vi "Dummy_Cam.vi"(4 "Frames in sequence":u32, 6 "Image in":variant, 7 "Camera-specific in":variant, 8 "Save path":path, 9 "Capture mode":enum16{"Single frame", "Sequence"}(ring), 10 "Exposure time (s)":dbl, 11 "Operation":T2(ring)) -> (3 "Status":T1, 5 "Camera-specific out":variant)   [LabVIEW 2015]
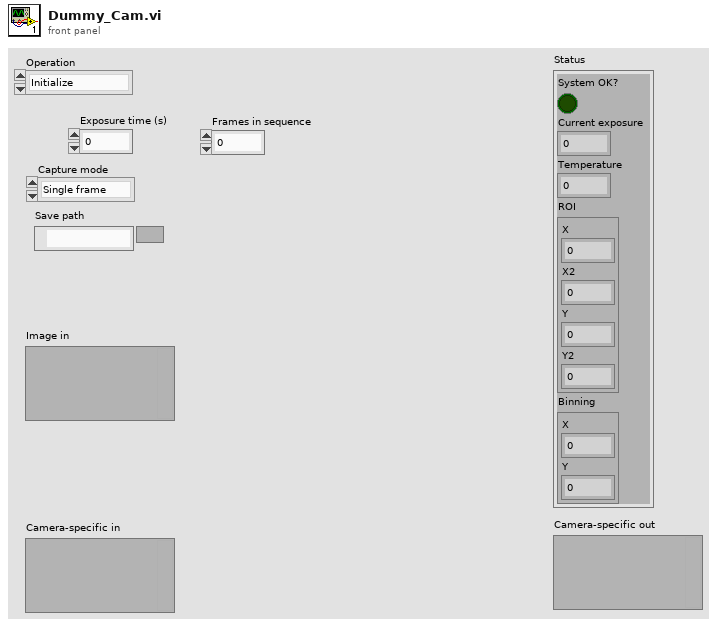
[diagram p1: front panel]
types:
  T1 = cluster{"System OK?":bool, "Current exposure":dbl, "Temperature":dbl, "ROI":cluster{"X":u32, "X2":u32, "Y":u32, "Y2":u32}, "Binning":cluster{"X":u32, "Y":u32}}
  T2 = enum16{"Initialize", "Shut down", "Set capture mode", "Set exposure", "Trigger and read", "Get status", "Other settings"}
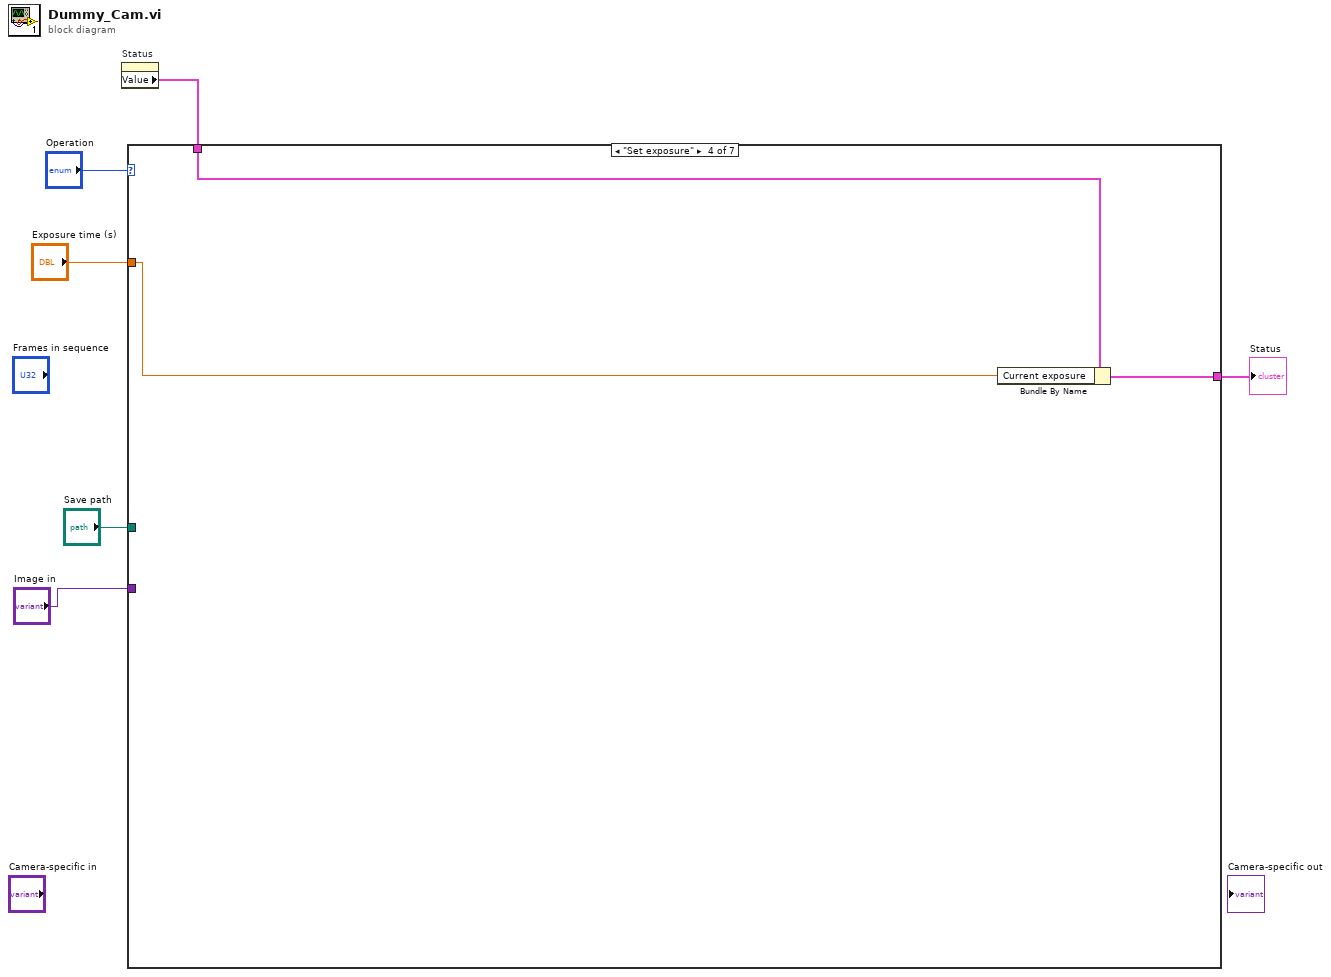
[diagram p0: block diagram]
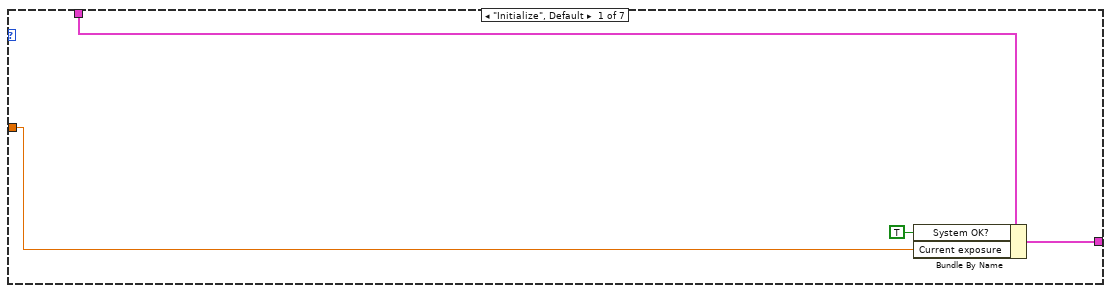
[diagram p2: hidden frame]
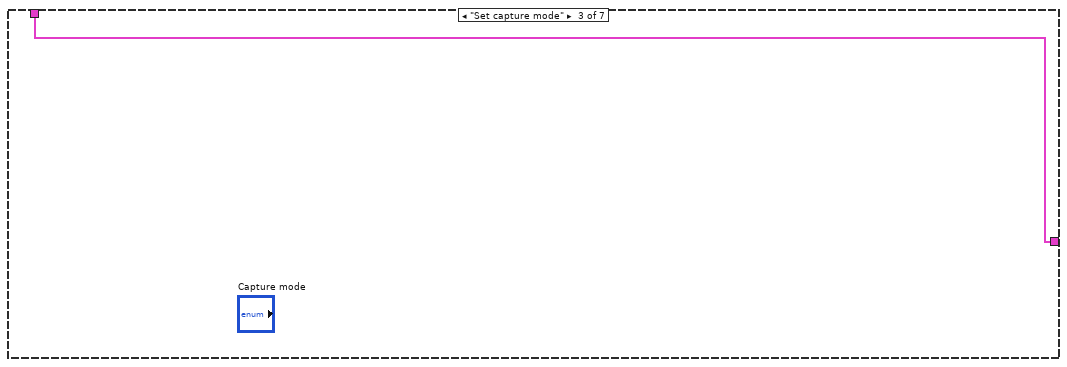
[diagram p4: hidden frame]
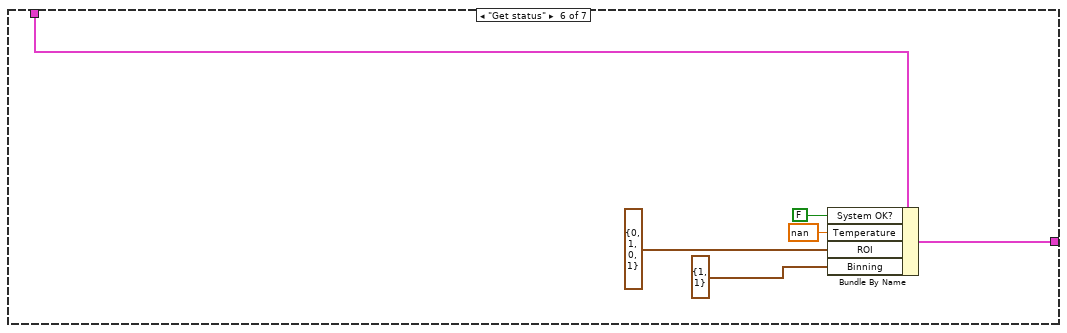
[diagram p6: hidden frame]
diagram:
  n1 = property on="Status" class="Clust (strict)"() -> ("Value"=w4:T1)  [unwired: 2 in, 2 out]
  n2 = case shown="\"Set exposure\"" "Operation" {
    tunnel: "Exposure time (s)" -> [w8 _ _ w13 _ _ _]
    tunnel: w4 -> [w10 w11 w12 w15 w16 w22 w23]
    tunnel: [w9 w11 w12 w14 w16 w21 w23] -> w3
    tunnel: "Save path" -> [_ _ _ _ _ _ _]
    tunnel: "Image in" -> [_ _ _ _ _ _ _]
    frame "Initialize", Default {
      n3 = Bundle By Name(cluster=w10, "System OK?"=TRUE, "Current exposure"=w8) -> (w9:T1)
    }
    frame "Shut down" {
    }
    frame "Set capture mode" {
    }
    frame "Set exposure" {
      n4 = Bundle By Name(cluster=w15, "Current exposure"=w13) -> (w14:T1)
    }
    frame "Trigger and read" {
    }
    frame "Get status" {
      n5 = Bundle By Name(cluster=w22, "System OK?"=FALSE, "Temperature"=nan, "ROI"=cluster{"X":u32, "X2":u32, "Y":u32, "Y2":u32} {"X"=0, "X2"=1, "Y"=0, "Y2"=1}, "Binning"=cluster{"X":u32, "Y":u32} {"X"=1, "Y"=1}) -> (w21:T1)
    }
    frame "Other settings" {
    }
  }
  "Status" <- w3
